vi "RT_MPU9250_postprocess_subVI_rev1.vi"(0 "readings in bits":bool[](array[boolean]), 1 "number of samples":i32) -> (6 "ZCompass":dbl, 7 "Zgyro":dbl, 8 "readings in decimal":u32[](array[numeric]), 9 "Ygyro":dbl, 10 "XAccel":dbl, 11 "Gyroscope (deg/s)":cluster{dbl, dbl, dbl}(graph), 12 "YCompass":dbl, 13 "Xgyro":dbl, 14 "Acceleration (g)":cluster{dbl, dbl, dbl}(graph), 15 "Compass":cluster{dbl, dbl, dbl}(graph), 16 "YAccel":dbl, 17 "XCompass":dbl, 18 "ZAccel":dbl)   [LabVIEW 2015]
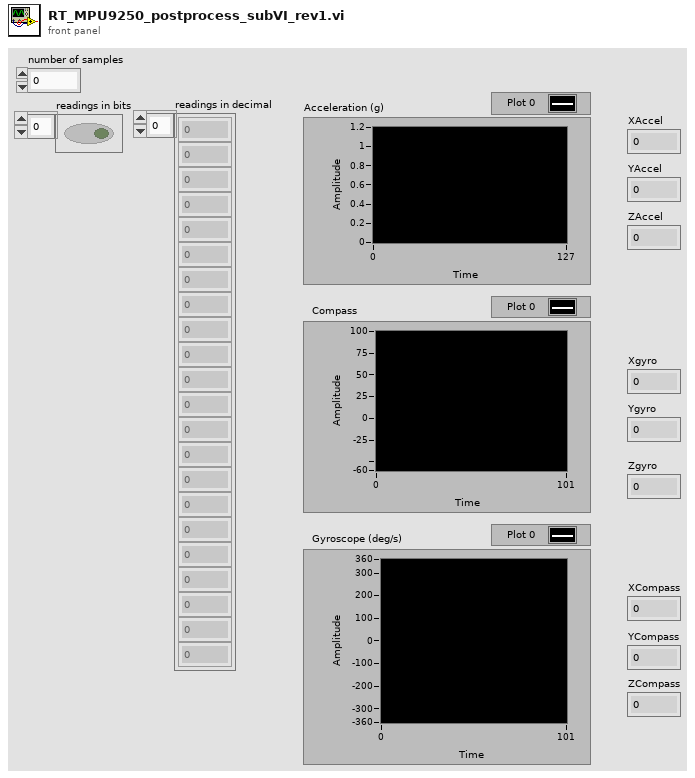
[diagram p1: front panel]
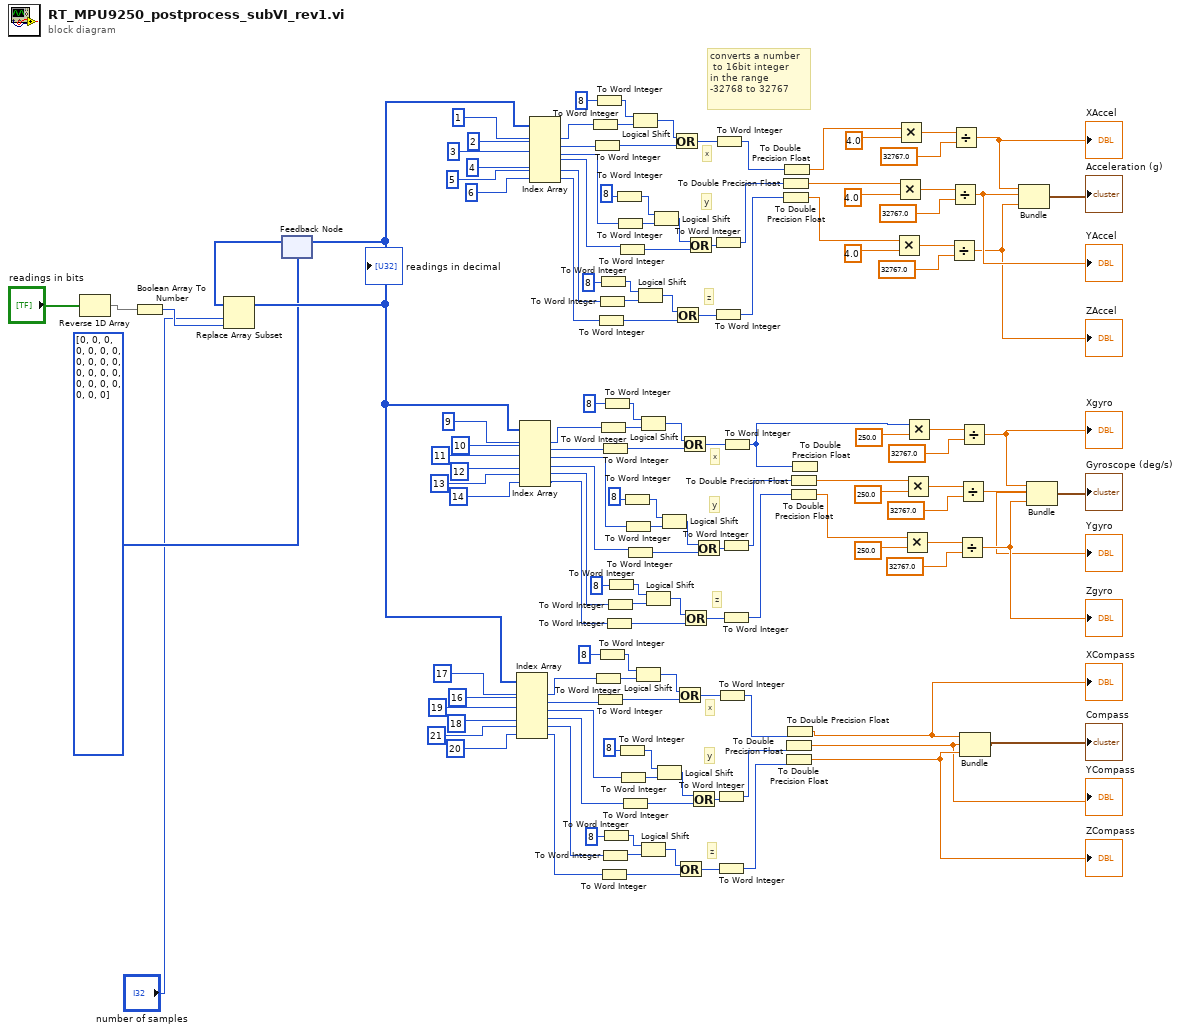
[diagram p0: block diagram]
diagram:
  # "z"
  # "y"
  # "x"
  # "z"
  # "y"
  # "x"
  # "converts a number\n to 16bit integer \nin the range \n-32768 to 32767"
  # "z"
  # "y"
  # "x"
  n1 = Reverse 1D Array(array="readings in bits") -> (reversed array=w59:bool[])
  n2 = Boolean Array To Number ("Boolean Array\n To Number")(Boolean array=w59) -> (number=w45:u32)
  n3 = feedback #1(u32[] [0, 0, 0, 0, 0, 0, 0, 0, 0, 0, 0, 0, 0, 0, 0, 0, 0, 0, 0, 0, 0, 0] ("array")) -> (w140:u32[])
  "readings in decimal" <- w140
  n4 = Replace Array Subset(array=w140, new element=w45, index="number of samples") -> (w46:u32[])
  n5 = feedback-in #1(w46) -> ()
  n6 = Index Array(array=w140, index #1=17 ("index"), index #2=16 ("index"), index #3=19 ("index"), index #4=18 ("index"), index #5=21 ("index"), index #6=20 ("index")) -> (element #1=w127:u32, element #2=w139:u32, element #3=w128:u32, element #4=w129:u32, element #5=w130:u32, element #6=w131:u32)
  n7 = Index Array(array=w140, index #1=9 ("index"), index #2=10 ("index"), index #3=11 ("index"), index #4=12 ("index"), index #5=13 ("index"), index #6=14 ("index")) -> (element #1=w101:u32, element #2=w100:u32, element #3=w102:u32, element #4=w103:u32, element #5=w104:u32, element #6=w105:u32)
  n8 = Index Array "Index Array"(array=w140, index #1=1 ("index"), index #2=2 ("index"), index #3=3 ("index"), index #4=4 ("index"), index #5=5 ("index"), index #6=6 ("index")) -> (element #1=w15:u32, element #2=w20:u32, element #3=w31:u32, element #4=w35:u32, element #5=w40:u32, element #6=w64:u32)
  n9 = To Word Integer(number=w15) -> (16bit integer=w16:i16)
  n10 = To Word Integer(number=w20) -> (16bit integer=w19:i16)
  n11 = To Word Integer(number=w127) -> (16bit integer=w110:i16)
  n12 = To Word Integer(number=i16 8 ("y")) -> (16bit integer=w17:i16)
  n13 = To Word Integer(number=w139) -> (16bit integer=w113:i16)
  n14 = To Word Integer(number=w64) -> (16bit integer=w63:i16)
  n15 = To Word Integer(number=w40) -> (16bit integer=w39:i16)
  n16 = To Word Integer(number=i16 8 ("y")) -> (16bit integer=w111:i16)
  n17 = To Word Integer(number=i16 8 ("y")) -> (16bit integer=w38:i16)
  n18 = To Word Integer(number=w101) -> (16bit integer=w70:i16)
  n19 = To Word Integer(number=w131) -> (16bit integer=w126:i16)
  n20 = To Word Integer(number=w100) -> (16bit integer=w73:i16)
  n21 = To Word Integer(number=w130) -> (16bit integer=w120:i16)
  n22 = To Word Integer(number=i16 8 ("y")) -> (16bit integer=w119:i16)
  n23 = To Word Integer(number=i16 8 ("y")) -> (16bit integer=w71:i16)
  n24 = To Word Integer(number=w105) -> (16bit integer=w98:i16)
  n25 = To Word Integer(number=w104) -> (16bit integer=w90:i16)
  n26 = To Word Integer(number=i16 8 ("y")) -> (16bit integer=w89:i16)
  n27 = To Word Integer(number=i16 8 ("y")) -> (16bit integer=w33:i16)
  n28 = To Word Integer(number=w31) -> (16bit integer=w34:i16)
  n29 = To Word Integer(number=w35) -> (16bit integer=w36:i16)
  n30 = To Word Integer(number=i16 8 ("y")) -> (16bit integer=w115:i16)
  n31 = To Word Integer(number=w128) -> (16bit integer=w116:i16)
  n32 = To Word Integer(number=w129) -> (16bit integer=w117:i16)
  n33 = To Word Integer(number=i16 8 ("y")) -> (16bit integer=w85:i16)
  n34 = To Word Integer(number=w102) -> (16bit integer=w86:i16)
  n35 = To Word Integer(number=w103) -> (16bit integer=w87:i16)
  n36 = Logical Shift(y=w17, x=w16) -> (x << y=w10:i16)
  n37 = Logical Shift(y=w111, x=w110) -> (x << y=w106:i16)
  n38 = Logical Shift(y=w38, x=w39) -> (x << y=w43:i16)
  n39 = Logical Shift(y=w71, x=w70) -> (x << y=w65:i16)
  n40 = Logical Shift(y=w119, x=w120) -> (x << y=w122:i16)
  n41 = Logical Shift(y=w89, x=w90) -> (x << y=w92:i16)
  n42 = Logical Shift(y=w33, x=w34) -> (x << y=w11:i16)
  n43 = Logical Shift(y=w115, x=w116) -> (x << y=w107:i16)
  n44 = Logical Shift(y=w85, x=w86) -> (x << y=w66:i16)
  n45 = Or(x=w10, y=w19) -> (x .or. y?=w13:i16)
  n46 = Or(x=w43, y=w63) -> (x .or. y?=w42:i16)
  n47 = Or(x=w106, y=w113) -> (x .or. y?=w108:i16)
  n48 = Or(x=w122, y=w126) -> (x .or. y?=w121:i16)
  n49 = Or(x=w65, y=w73) -> (x .or. y?=w68:i16)
  n50 = Or(x=w92, y=w98) -> (x .or. y?=w91:i16)
  n51 = Or(x=w11, y=w36) -> (x .or. y?=w14:i16)
  n52 = Or(x=w107, y=w117) -> (x .or. y?=w109:i16)
  n53 = Or(x=w66, y=w87) -> (x .or. y?=w69:i16)
  n54 = To Word Integer(number=w14) -> (16bit integer=w137:i16)
  n55 = To Word Integer(number=w42) -> (16bit integer=w138:i16)
  n56 = To Word Integer(number=w13) -> (16bit integer=w136:i16)
  n57 = To Word Integer(number=w109) -> (16bit integer=w125:i16)
  n58 = To Word Integer(number=w121) -> (16bit integer=w124:i16)
  n59 = To Word Integer(number=w108) -> (16bit integer=w123:i16)
  n60 = To Word Integer(number=w69) -> (16bit integer=w97:i16)
  n61 = To Word Integer(number=w91) -> (16bit integer=w93:i16)
  n62 = To Word Integer(number=w68) -> (16bit integer=w1:i16)
  n63 = To Double Precision Float(number=w137) -> (double precision float=w29:dbl)
  n64 = To Double Precision Float(number=w138) -> (double precision float=w30:dbl)
  n65 = To Double Precision Float(number=w136) -> (double precision float=w41:dbl)
  n66 = To Double Precision Float(number=w125) -> (double precision float=w133:dbl)
  "YCompass" <- w133
  n67 = To Double Precision Float(number=w124) -> (double precision float=w134:dbl)
  "ZCompass" <- w134
  n68 = To Double Precision Float(number=w123) -> (double precision float=w132:dbl)
  "XCompass" <- w132
  n69 = To Double Precision Float(number=w97) -> (double precision float=w82:dbl)
  n70 = To Double Precision Float(number=w93) -> (double precision float=w83:dbl)
  n71 = To Double Precision Float(number=w1) -> ()  [unwired: 1 out]
  n72 = Multiply(x=w30, y=4.0) -> (x*y=w26:dbl)
  n73 = Multiply(x=w29, y=4.0) -> (x*y=w25:dbl)
  n74 = Multiply(x=w41, y=4.0) -> (x*y=w12:dbl)
  n75 = Multiply(x=w83, y=250.0) -> (x*y=w79:dbl)
  n76 = Multiply(x=w82, y=250.0) -> (x*y=w78:dbl)
  n77 = Multiply(x=w1, y=250.0) -> (x*y=w67:dbl)
  n78 = Divide(x=w26, y=32767.0) -> (x/y=w62:dbl)
  "ZAccel" <- w62
  n79 = Divide(x=w25, y=32767.0) -> (x/y=w141:dbl)
  "YAccel" <- w141
  n80 = Divide(x=w12, y=32767.0) -> (x/y=w61:dbl)
  "XAccel" <- w61
  n81 = Divide(x=w79, y=32767.0) -> (x/y=w96:dbl)
  "Zgyro" <- w96
  n82 = Divide(x=w78, y=32767.0) -> (x/y=w95:dbl)
  "Ygyro" <- w95
  n83 = Divide(x=w67, y=32767.0) -> (x/y=w94:dbl)
  "Xgyro" <- w94
  n84 = Bundle(w132, w133, w134) -> (→"Compass":cluster{dbl, dbl, dbl})  [unwired: 1 in]
  n85 = Bundle(w61, w141, w62) -> (→"Acceleration (g)":cluster{dbl, dbl, dbl})  [unwired: 1 in]
  n86 = Bundle(w94, w95, w96) -> (→"Gyroscope (deg/s)":cluster{dbl, dbl, dbl})  [unwired: 1 in]
